vi "ValidateInputs.vi"(8 "error in (no error)":errorcluster, 11 "RunTests in":refnum<class "RunVITester.lvclass">) -> (0 "error out":errorcluster, 3 "RunTests out":refnum<class "RunVITester.lvclass">)   [LabVIEW 2027, in "RunVITester.lvclass"]
uses:
  RunVITester.lvclass
  RunVITester.lvclass/RunVITester.ctl
  <nishared>/LabVIEW CLI/Operations/Utilities/OperationErrorType.ctl
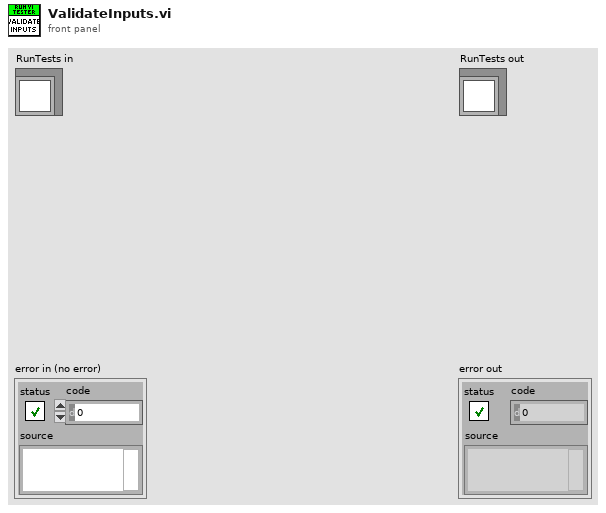
[diagram p1: front panel]
types:
  T1 = typedef "OperationErrorType.ctl" = enum16{"RequiredArgumentMissing", "UnknownArguments", "LoggerSetMultipleTimes", "OperationBrokenError"}
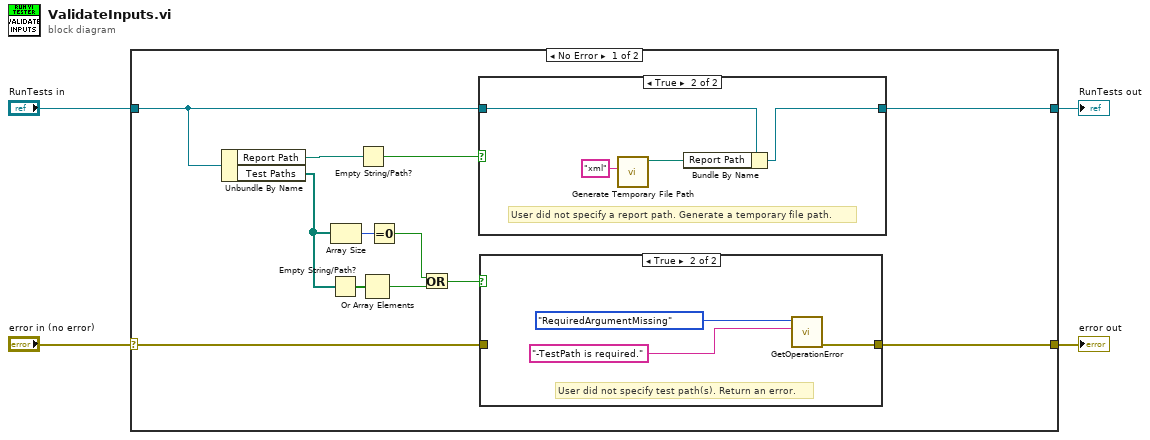
[diagram p0: block diagram]
diagram:
  n1 = case shown="No Error" "error in (no error)" {
    selector: "error in (no error)" -> [w14 w27]
    tunnel: [w15 w27] -> w3
    tunnel: [w10 w26] -> w1
    tunnel: "RunTests in" -> [w11 w26]
    frame No Error {
      n2 = Unbundle By Name(w11) -> ("Report Path"=w13:path, "Test Paths"=w9:path[])
      n3 = Empty String/Path?(string/path=w9) -> (empty?=w16:bool[])
      n4 = Array Size(array=w9) -> (size(s)=w7:i32)
      n5 = Empty String/Path?(string/path=w13) -> (empty?=w12:bool)
      n6 = Or Array Elements(Boolean array=w16) -> (logical OR=w8:bool)
      n7 = Equal To 0?(x=w7) -> (x = 0?=w6:bool)
      n8 = Or(x=w6, y=w8) -> (x .or. y?=w5:bool)
      n9 = case shown="True" w12 {
        tunnel: w11 -> [w17 w21]
        tunnel: [w17 w20] -> w10
        frame False {
        }
        frame True {
          # "User did not specify a report path. Generate a temporary file path."
          n10 = call <vilib>:"Generate Temporary File Path.vi"("Temporary File Extension (tmp)"="xml") -> ("Unique Temporary File Path"=w18:path)  [unwired: 9 in, 1 out]
          n11 = Bundle By Name(cluster=w21, "Report Path"=w18) -> (w20:refnum<class "RunVITester.lvclass">)
        }
      }
      n12 = case shown="True" w5 {
        tunnel: [w22 w25] -> w15
        tunnel: w14 -> [w22 _]
        frame False {
        }
        frame True {
          # "User did not specify test path(s). Return an error."
          n13 = call <nishared>:"GetOperationError.vi"("Additional Information"="-TestPath is required.", "Operation Error Type"=OperationErrorType."RequiredArgumentMissing") -> ("error out"=w25:errorcluster)  [unwired: 9 in]
        }
      }
    }
    frame Error {
    }
  }
  "error out" <- w3
  "RunTests out" <- w1
